vi "WaterTankEU.vi"() -> ()   [LabVIEW 2021]
panel:
  out "Numeric":dbl
  in  "stop":bool
  out "Tank":dbl(slide) scale=0.0..20.0
  in  "Voltage":dbl(slide) scale=0.0..5.0
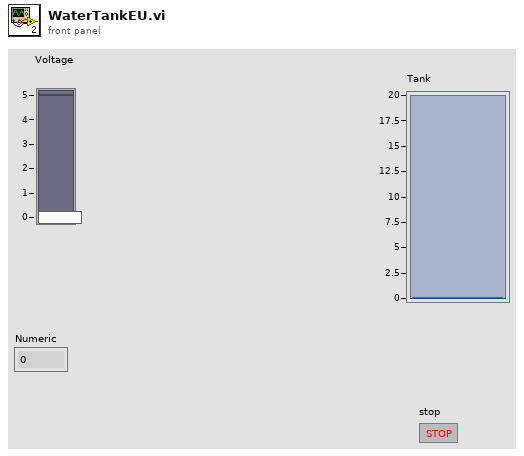
[diagram p1: front panel]
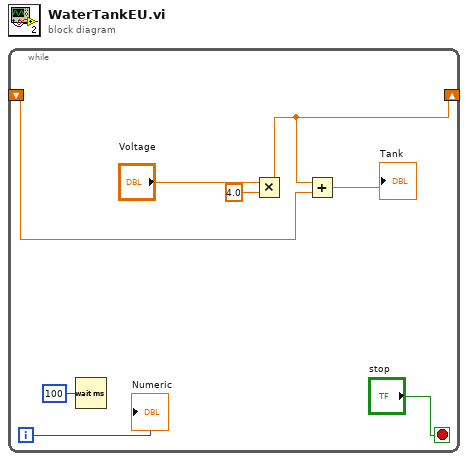
[diagram p0: block diagram]
diagram:
  n1 = while {
    shift-right: [w3] -> _
    shift-left: _ -> [w2]
    i -> [w4]
    stop <- "stop" stop-if-true
    n2 = Wait (ms)(milliseconds to wait=u32 100) -> ()  [unwired: 1 out]
    n3 = Multiply(x="Voltage", y=4.0) -> (x*y=w3:dbl)
    n4 = Add(x=w3, y=w2) -> (x+y=→"Tank":dbl)
    "Numeric" <- w4
  }
